vi "ConvertVoltToDegree2.vi"(10 "Tension":dbl) -> (2 "Température":dbl)   [LabVIEW 2022 SP3]
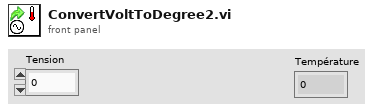
[diagram p1: front panel]
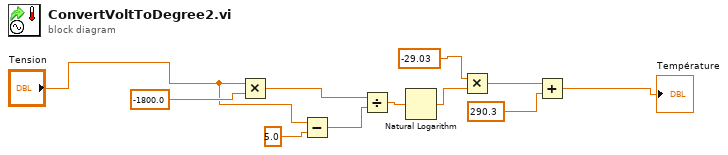
[diagram p0: block diagram]
diagram:
  n1 = Multiply(x="Tension", y=-1800.0) -> (x*y=w10:dbl)
  n2 = Subtract(x="Tension", y=5.0 ("x")) -> (x-y=w3:dbl)
  n3 = Divide(x=w10, y=w3) -> (x/y=w9:dbl)
  n4 = Natural Logarithm(1:w9) -> (0:w8:dbl)
  n5 = Multiply(x=-29.03, y=w8) -> (x*y=w7:dbl)
  n6 = Add(x=w7, y=290.3 ("x")) -> (x+y=→"Température":dbl)
